vi "18_ВПИзвлечениеКвадратногоКорня.vi"() -> ()   [LabVIEW 2016]
panel:
  out "Square Root Value":dbl
  in  "Number":dbl
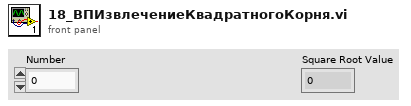
[diagram p1: front panel]
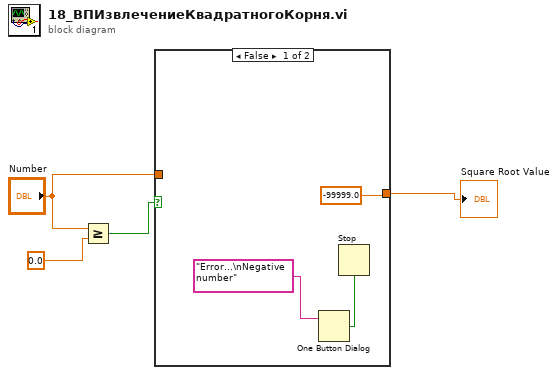
[diagram p0: block diagram]
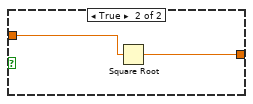
[diagram p2: hidden frame]
diagram:
  n1 = Greater Or Equal?(x="Number", y=0.0) -> (x >= y?=w3:bool)
  n2 = case shown="False" w3 {
    tunnel: "Number" -> [_ w9]
    tunnel: [-99999.0 w8] -> w1
    frame False {
      n3 = One Button Dialog(message="Error...\nNegative number") -> (true=w5:bool)  [unwired: 1 in]
      n4 = Stop(stop? (T)=w5) -> ()
    }
    frame True {
      n5 = Square Root(x=w9) -> (sqrt(x)=w8:dbl)
    }
  }
  "Square Root Value" <- w1
